vi "air flow valve controller (source sensor).vi"(4 "State":i16, 5 "Time":dbl format="%.2f", 6 "Sensor Values":dbl[](array[numeric])=[120000.0, 10000.0], 7 "Set Points":dbl[](array[numeric])=[1.0, 22.0, 5e-05]) -> (0 "required data":T1={"Set Point names"=["slope (s^-1 m^-1 mol^-1 kg)", "air flow (M/s)"], "required number of setpoints"=2, "required number of sensors"=2, "Sensor names"=["Accumulator pressure (Pa)", "Source pressure (Pa)"]}, 3 "fraction on":dbl)   [LabVIEW 2015]
panel:
  # "Enter the correct information for this control code in the required data structure below. Then make the current value default by right clicking on the border of the data structure."
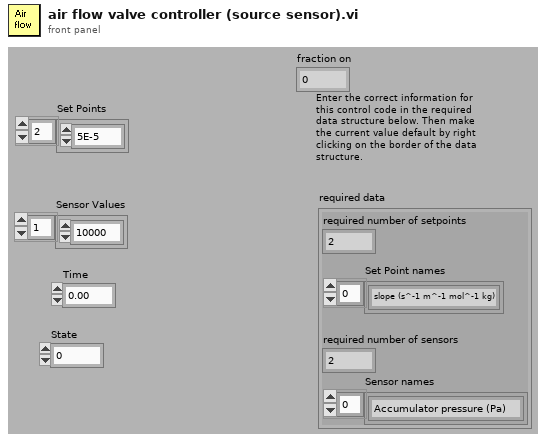
[diagram p1: front panel]
types:
  T1 = cluster{"Set Point names":string[], "required number of setpoints":u8, "required number of sensors":u8, "Sensor names":string[]}
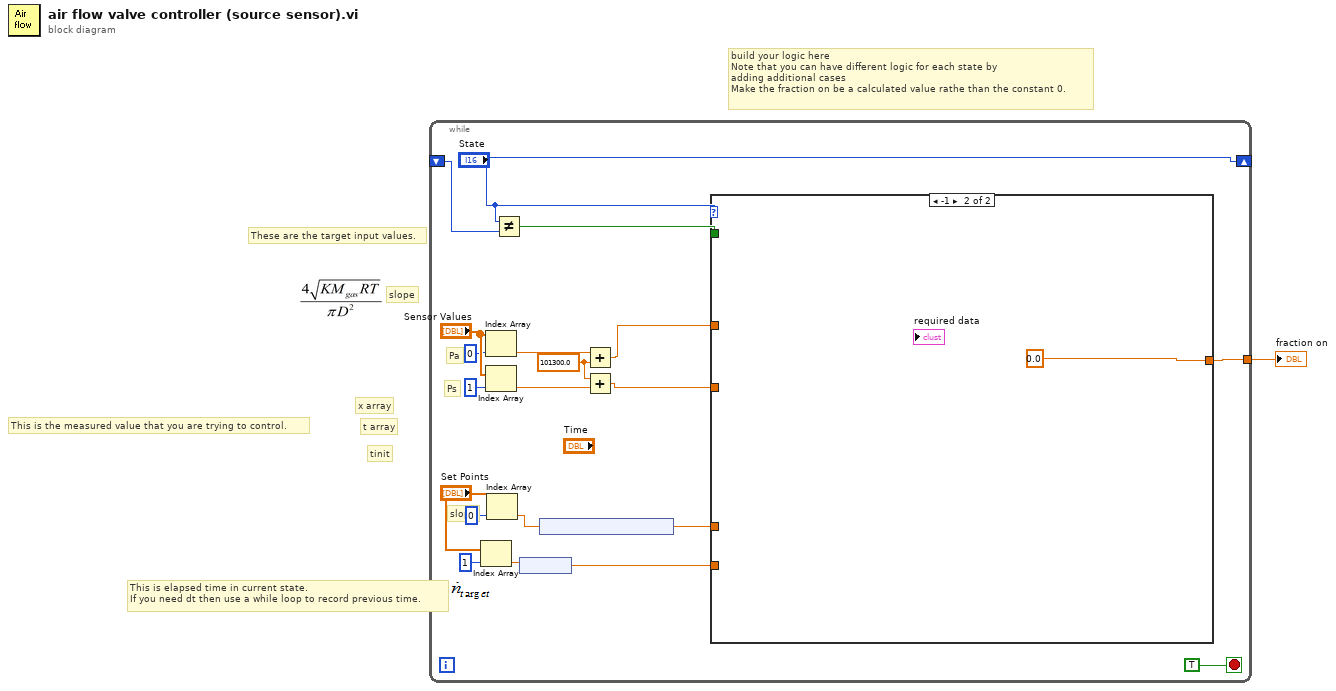
[diagram p0: block diagram]
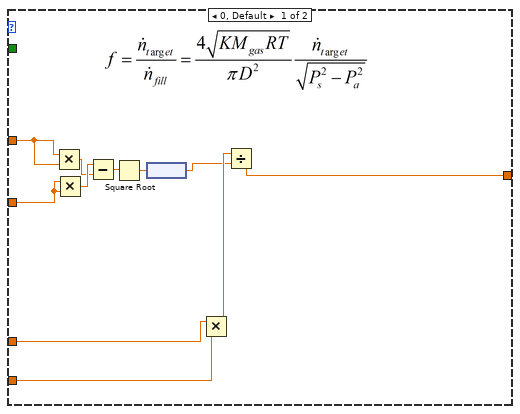
[diagram p2: hidden frame]
diagram:
  # "slope"
  # "tinit"
  # "t array"
  # "x array"
  # "build your logic here\nNote that you can have different logic for each state by\nadding additional cases\nMake the fraction on be a calculated value rathe than the constant 0."
  # "These are the target input values."
  # "This is the measured value that you are trying to control."
  # "This is elapsed time in current state.\nIf you need dt then use a while loop to record previous time."
  n1 = while {
    tunnel: [w21] -> w1
    shift-right: ["State"] -> _
    shift-left: _ -> [w17]
    stop <- TRUE stop-if-true
    w4 = 101300.0 ("y")
    # "slope"
    # "Ps"
    # "Pa"
    n2 = Index Array(array="Set Points", index=1) -> (element=w11:dbl)
    n3 = Index Array(array="Sensor Values", index=0) -> (element=w8:dbl)
    n4 = Index Array(array="Sensor Values", index=1) -> (element=w7:dbl)
    n5 = Index Array(array="Set Points", index=0) -> (element=w3:dbl)
    n6 = Not Equal?(x="State", y=w17) -> (x != y?=w15:bool)
    n7 = node(w11) -> (w10:dbl[unit])
    n8 = node(w3) -> (w2:dbl[unit])
    n9 = Add(x=w8, y=w4) -> (x+y=w5:dbl)
    n10 = Add(x=w4, y=w7) -> (x+y=w6:dbl)
    n11 = case shown="-1" "State" {
      tunnel: [w23 0.0 ("fraction on")] -> w21
      tunnel: w15 -> [_ _]
      tunnel: w10 -> [w32 _]
      tunnel: w5 -> [w31 _]
      tunnel: w6 -> [w30 _]
      tunnel: w2 -> [w22 _]
      frame 0, Default {
        n12 = Multiply(x=w31, y=w31) -> (x*y=w28:dbl)
        n13 = Multiply(x=w30, y=w30) -> (x*y=w29:dbl)
        n14 = Subtract(x=w29, y=w28) -> (x-y=w27:dbl)
        n15 = Square Root(x=w27) -> (sqrt(x)=w26:dbl)
        n16 = node(w26) -> (w24:dbl[unit])
        n17 = Multiply(x=w22, y=w32) -> (x*y=w25:dbl[unit])
        n18 = Divide(x=w25, y=w24) -> (x/y=w23:dbl)
      }
      frame -1 {
      }
    }
  }
  "fraction on" <- w1
